vi "Read Radio.vi"(8 "error in (no error)":errorcluster, 11 "Circulo in":refnum<class "Circulo.lvclass">) -> (0 "error out":errorcluster, 2 "Radio":dbl, 3 "Circulo out":refnum<class "Circulo.lvclass">)   [LabVIEW 2024, in "Circulo.lvclass"]
uses:
  Circulo.lvclass
  Circulo.lvclass/Circulo.ctl
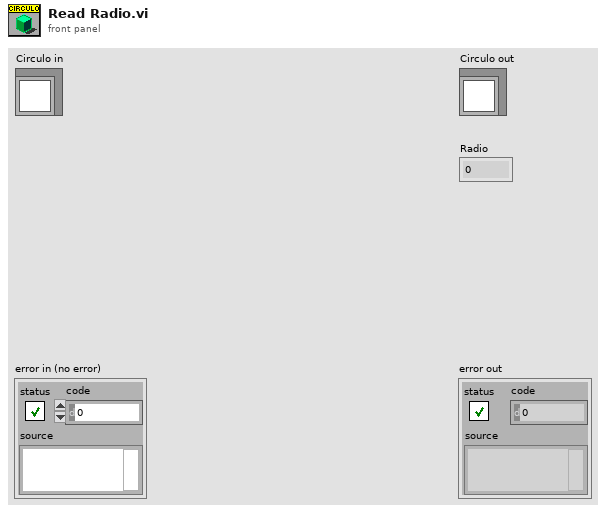
[diagram p1: front panel]
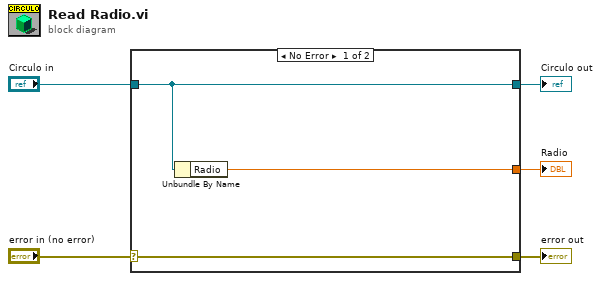
[diagram p0: block diagram]
diagram:
  n1 = case shown="No Error" "error in (no error)" {
    selector: "error in (no error)" -> [w8 w9]
    tunnel: [w8 w9] -> w4
    tunnel: [w7 w10] -> w2
    tunnel: "Circulo in" -> [w7 w10]
    tunnel: [w6 _] -> w1
    frame No Error {
      n2 = Unbundle By Name(w7) -> ("Radio"=w6:dbl)
    }
    frame Error {
    }
  }
  "error out" <- w4
  "Circulo out" <- w2
  "Radio" <- w1
